vi "EasyFlux.vi"() -> ()   [LabVIEW 2017]
uses:
  Types/EF_GUIThread_SMCmds.ctl
  Types/EF_GUIThread_QData.ctl
  Types/EF_GUIThread_QCmds.ctl
  Types/EF_DAQThread_QData.ctl
  Types/EF_DAQThread_QCmds.ctl
  Types/EF_DataProcThread_QData.ctl
  Types/EF_DataProcThread_QCmds.ctl
  Types/EF_AnalysisThread_QData.ctl
  Types/EF_AnalysisThread_QCmds.ctl
panel:
  out "DeltaT":dbl caption="Resol.     ms" format="%.2f"
  in  "BitShift":i32 min=0 max=32 step=1
  in  "Threshold":i32 caption="Thresh. cnts" min=0 max=100000 step=1
  out "TimeChart":cluster{dbl, "DeltaT":dbl, u32[]}(graph)={0.0, "DeltaT"=0.0016383737860194236, []}
  in  "MinIntCounts":u32=1 caption="Min. Counts" min=1 step=1
  in  "DecayT0":dbl caption="DecayT0  ns" min=0.0 step=0.001
  in  "Offset":i32 caption="Offset      ps" min=0 max=100000 step=1
  in  "Binning":i32(ring) caption="Resol.      ps" items=["4", "8", "16", "32", "64", "128", "256", "512"]
  in  "CFD1 ZeroX":i32=10 caption="ZeroCr.  mV" min=0 max=20 step=1
  in  "CFD1 Level":i32=50 caption="Discr.     mV" min=0 max=800 step=1
  in  "Ch0 Divider":i32(ring)=1 caption="Divider" items=["1"=1, "2"=2, "4"=4, "8"=8]
  in  "Ch0 Offset":i32 caption="Offset      ps" min=-99999 max=99999 step=1
  in  "CFD0 ZeroX":i32=10 caption="ZeroCr.  mV" min=0 max=20 step=1
  in  "CFD0 Level":i32=50 caption="Discr.     mV" min=0 max=800 step=1
  out "HistoGraph":cluster{dbl, "Res":dbl, "Histo":u32[]}(graph)
  out "Pending":i32
  out "ShortDelay":bool caption="Short Delay"
  out "MinDelay":dbl(slide) caption="Minimum Delay             ms" scale=200.0..300.0 scale format="%#.0f"
  in  "LTThreshold":dbl caption="Thresh.    ns" min=0.0 step=0.001
  in  "Activate":bool
  in  "TTLWidth":i32=1 caption="Width     ms" min=1 max=10000 step=1
  in  "TTLDelay":i32=50 caption="Delay      ms" min=10 max=10000 step=1
  in  "Start":bool
  out "LTGraph":cluster{dbl[], "AvgLTs":dbl[]}(graph)
  out "Ch1 Rate:":i32 caption="Input1 / cps" format="%.2e"
  out "Ch0 Rate:":i32 caption="Sync / cps" format="%.2e"
  out "Status":string
  # "Time Trace"
  # "Histogram"
  # "Inp.Chan 1"
  # "Inp.Chan 0 / Sync"
  # "TTL Pulse"
  # "Lifetimes"
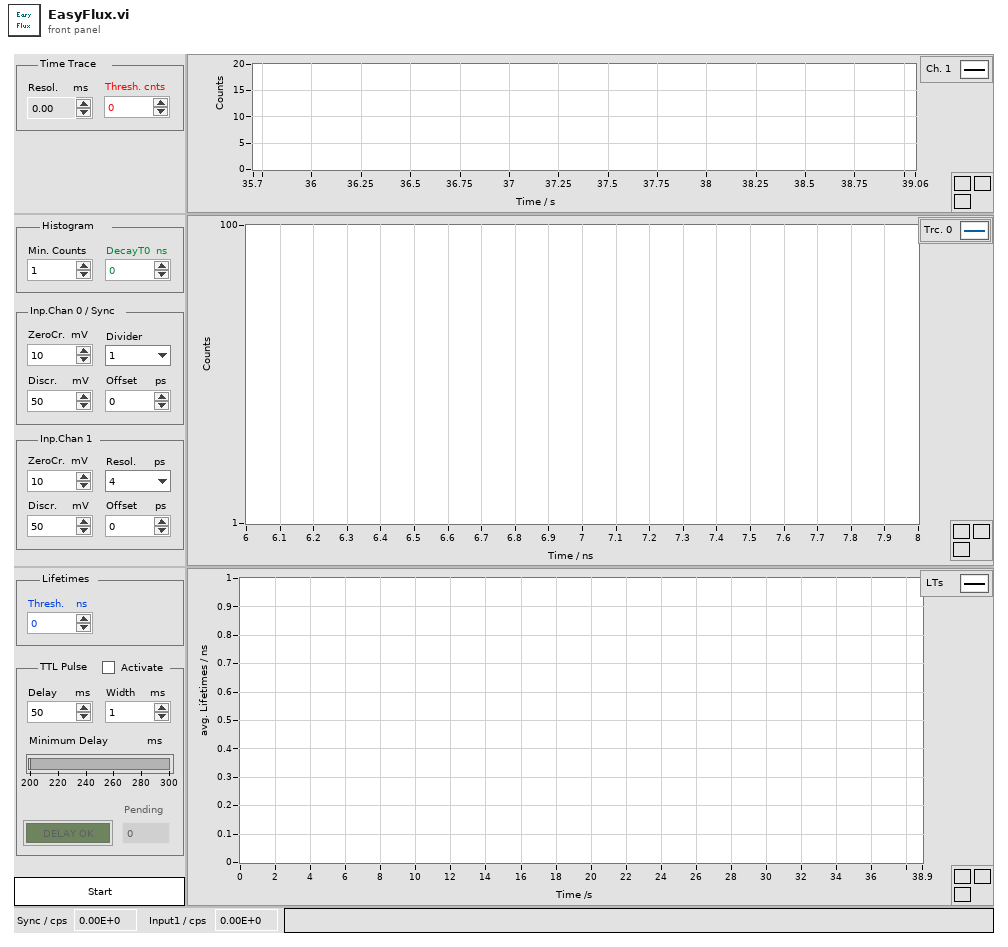
[diagram p1: front panel]
types:
  T1 = typedef "EF_GUIThread_QData.ctl" = cluster{"Histo":u32[], "Rates":i32[], "Cmd":T2, "Res":dbl, "TimeTrace":u32[], "Bin":i32, "Status":string, "Total bin":u64, "AvgLTs":dbl[], "TotalBinsHistStart":u64[], "HistStartTimes":dbl[], "MinDelays":dbl[], "ShortDelay":bool, "Pending TTLs":i32, "error in (no error)":errorcluster, "DeltaT":dbl, "NumLTs":i32}
  T2 = typedef "EF_GUIThread_QCmds.ctl" = enum16{"_none_", "Res", "Histo", "TTrace", "Lifetime", "Rates", "Status", "ShortDelay", "_Error_"}
  T3 = typedef "EF_GUIThread_SMCmds.ctl" = enum16{"Idle", "Enable Controls", "Init", "Timeout"}
  T4 = typedef "EF_GUIThread_IniData.ctl" = cluster{"Threshold":i32, "BitShift":i32, "DecayT0":dbl, "LTThreshold":dbl, "TTLDelay":i32, "TTLWidth":i32, "MinIntCounts":u32}
  T5 = typedef "EF_DAQThread_Data.ctl" = cluster{"LibraryVersion":string, "CFD0_Level":i32, "CFD0_ZeroX":i32, "CFD1_Level":i32, "CFD1_ZeroX":i32, "Ch0_Divider":i32, "Ch0_Offset":i32, "Init Info":T6, "DevIdx":i32, "Offset":i32, "Binning":i32, "Resolution":dbl, "DllPath":path, "Status":string}
  T6 = typedef "PH_InitInfo.ctl" = cluster{"Library Version":string, "Serial No.":string, "Model":string, "Partnum":string, "Version":string, "features":i32, "Base Resolution":dbl, "Bin Steps":i32, "DevIdx":i32}
  T7 = typedef "EF_AllQRefs.ctl" = cluster{"EF_GUIThread_QRef":T8, "EF_DAQThread_QRef":T9, "EF_DataProcThread_QRef":T10, "EF_AnalysisThread_QRef":T11}
  T8 = typedef "EF_GUIThread_QRef.ctl" = refnum<queue>
  T9 = typedef "EF_DAQThread_QRef.ctl" = refnum<queue>
  T10 = typedef "EF_DataProcThread_QRef.ctl" = refnum<queue>
  T11 = typedef "EF_AnalysisThread_QRef.ctl" = refnum<queue>
  T12 = typedef "EF_DAQThread_QData.ctl" = cluster{"EF_DAQThread_Cmds":T13, "Parameter":i32[], "error in (no error)":errorcluster}
  T13 = typedef "EF_DAQThread_QCmds.ctl" = enum16{"Idle", "Init", "InitHW", "SetCFD0", "SetCFD1", "SetCh0Divider", "SetCh0Offset", "SetOffset", "SetBinning", "GetResolution", "GetRates", "StartMeas", "ReadFiFo", "StopMeas", "WriteStatus", "_Error_", "Exit"}
  T14 = typedef "EF_DataProcThread_QCmds.ctl" = enum16{"Exit", "Proc", "Init", "SetShift", "SetThres"}
  T15 = typedef "EF_DataProcThread_QData.ctl" = cluster{"EF_DataProc_Cmds":T14, "nActual":i32, "Buffer":u32[], "TickCount":u32, "Param":i32}
  T16 = typedef "EF_AnalysisThread_QCmds.ctl" = enum16{"Exit", "CalcAvgLT", "CalcDelay", "SetDecayT0", "SetHistoRes", "SetTimeTraceRes", "SetLTThreshold", "SetTTLActiv", "SetTTLDelay", "SetTTLWidth", "SetMinIntCounts"}
  T17 = typedef "EF_AnalysisThread_QData.ctl" = cluster{"Cmd":T16, "Histo":u32[], "DecayT0":dbl, "HistoRes":dbl, "TotalBinHistStart":u64, "TimeTraceRes":dbl, "Total bin":u64, "TickCount":u32, "LTThreshold":dbl, "TTLActivate":bool, "TTLDelay":dbl, "TTLWidth":dbl, "MinIntCounts":u32}
  T18 = enum8{"Enabled", "Disabled", "Disabled and Grayed Out"}
  T19 = cluster{"T0":dbl, "dt":dbl, "TimeTrace_out":u32[]}
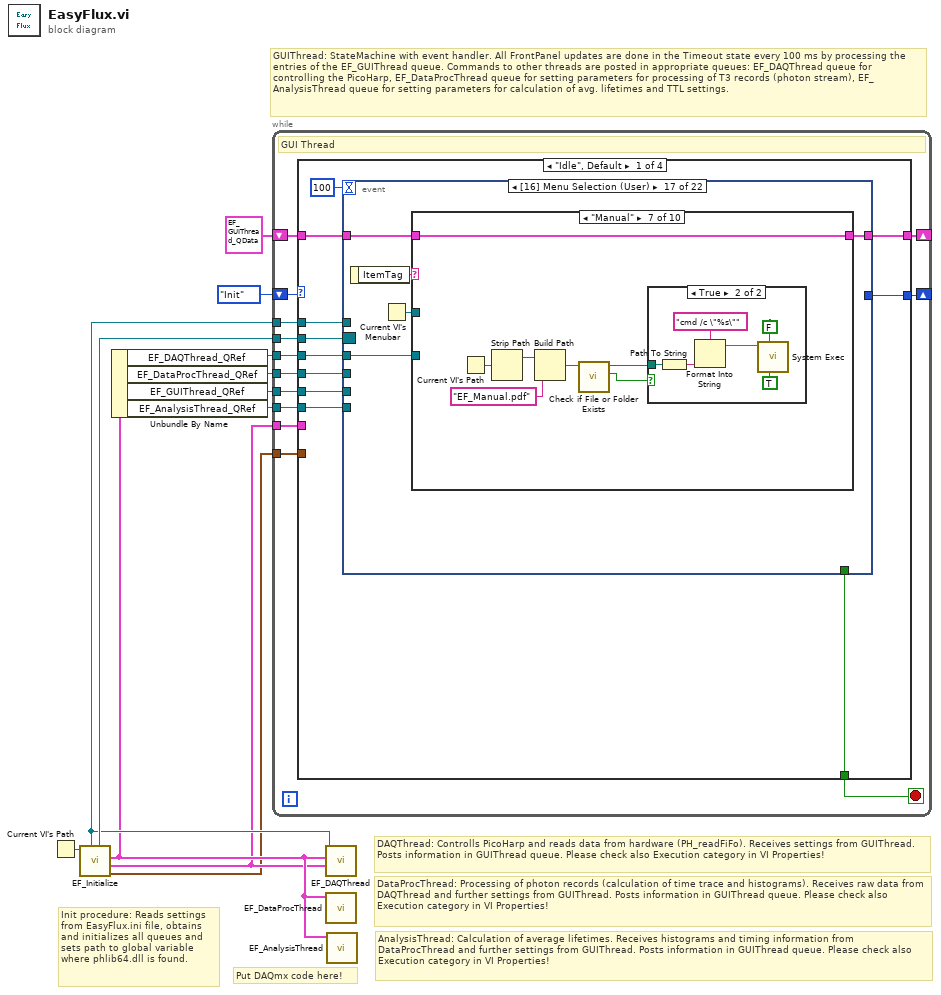
[diagram p0: block diagram]
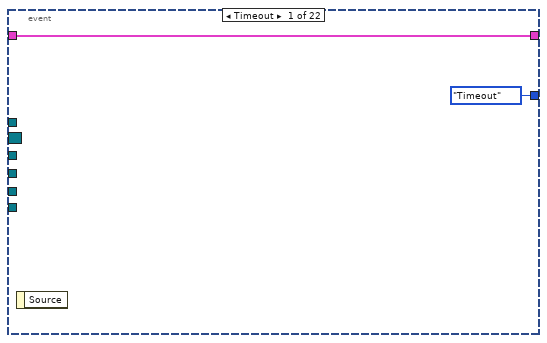
[diagram p2: hidden frame]
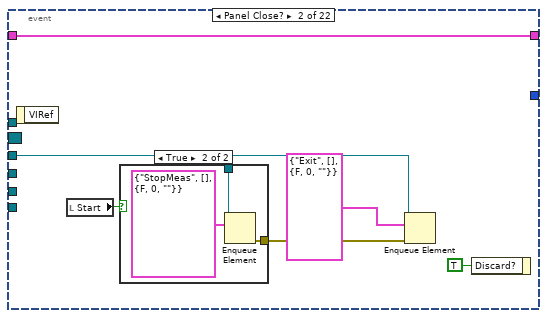
[diagram p3: hidden frame]
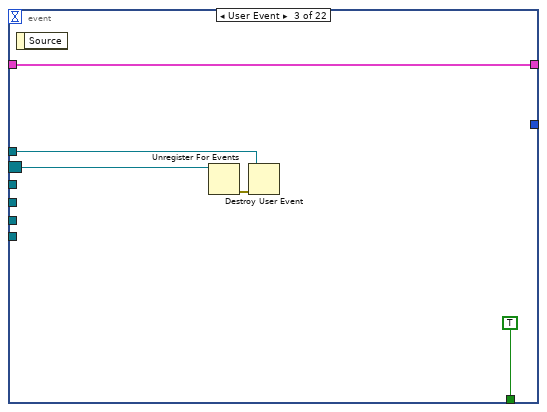
[diagram p5: hidden frame]
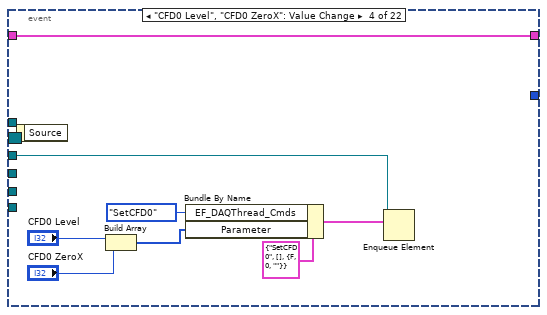
[diagram p6: hidden frame]
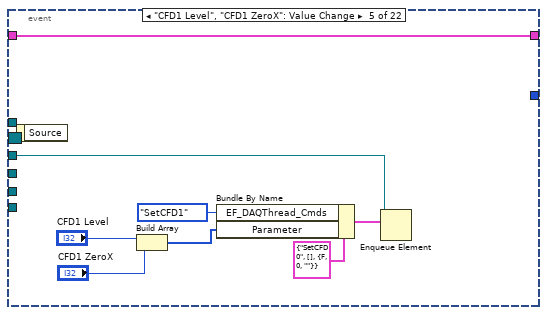
[diagram p7: hidden frame]
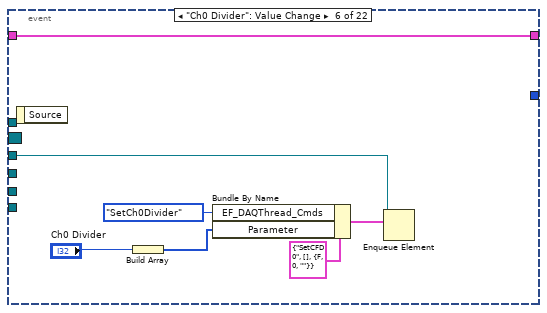
[diagram p8: hidden frame]
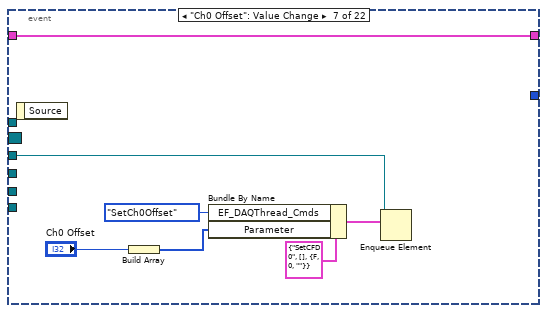
[diagram p9: hidden frame]
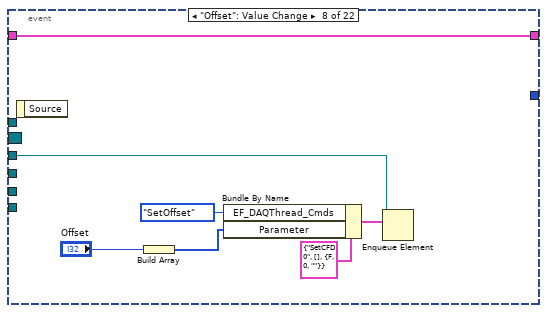
[diagram p10: hidden frame]
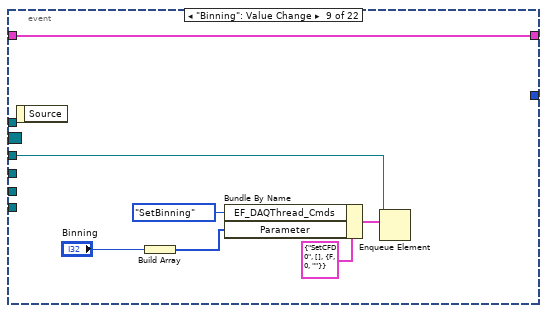
[diagram p11: hidden frame]
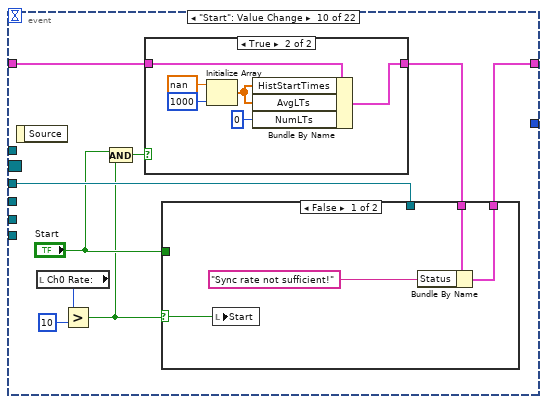
[diagram p12: hidden frame]
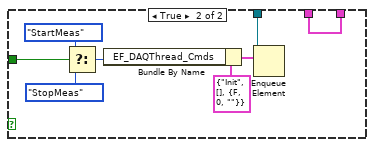
[diagram p13: hidden frame]
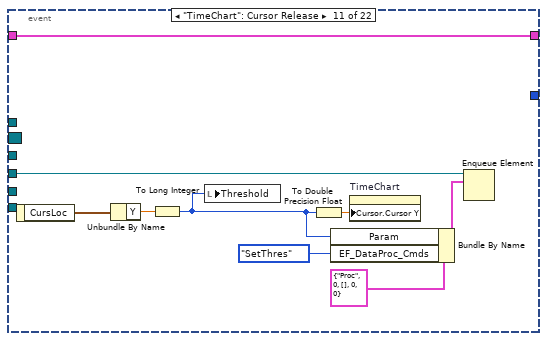
[diagram p15: hidden frame]
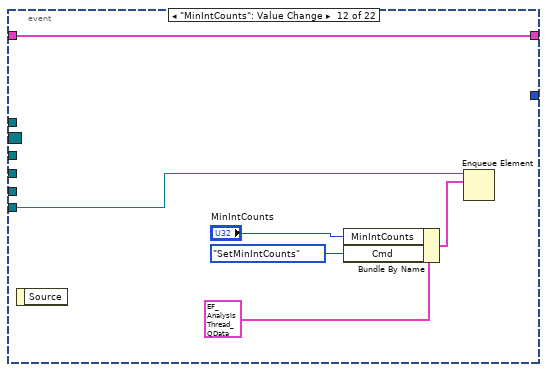
[diagram p16: hidden frame]
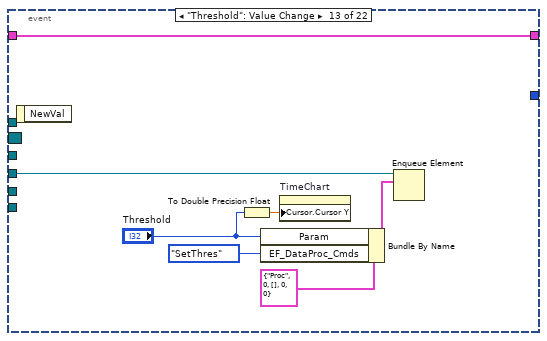
[diagram p17: hidden frame]
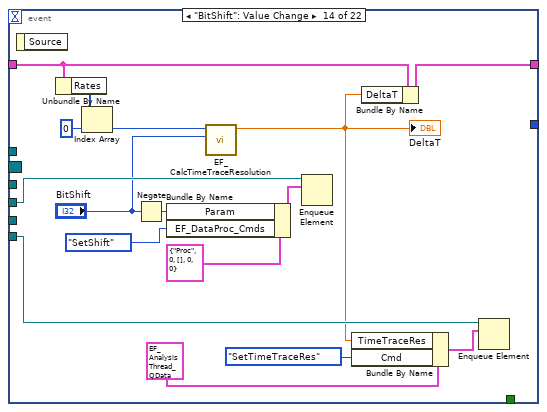
[diagram p18: hidden frame]
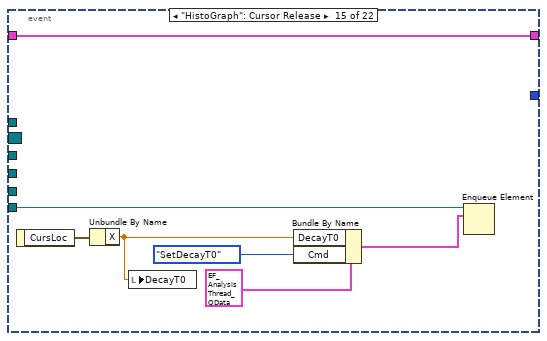
[diagram p19: hidden frame]
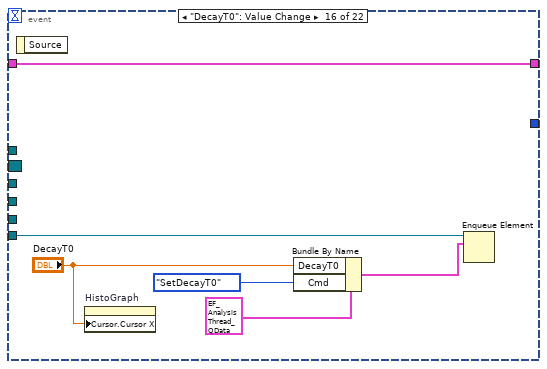
[diagram p20: hidden frame]
diagram:
  # "Init procedure: Reads settings from EasyFlux.ini file, obtains and initializes all queues and sets path to global variable where phlib64.dll is found."
  # "Put DAQmx code here!"
  # "DAQThread: Controlls PicoHarp and reads data from hardware (PH_readFiFo). Receives settings from GUIThread. Posts information in GUIThread queue. Please check also Execution category in VI Properties!"
  # "DataProcThread: Processing of photon records (calculation of time trace and histograms). Receives raw data from DAQThread and further settings from GUIThread. Posts information in GUIThread queue. Please check also Execution category in VI Properties!"
  # "GUIThread: StateMachine with event handler. All FrontPanel updates are done in the Timeout state every 100 ms by processing the entries of the EF_GUIThread queue. Commands to other threads are posted in appropriate queues: EF_DAQThread queue for controlling the PicoHarp, EF_DataProcThread queue for setting parameters for processing of T3 records (photon stream), EF_AnalysisThread queue for setting parameters for calculation of avg. lifetimes and TTL settings."
  # "AnalysisThread: Calculation of average lifetimes. Receives histograms and timing information from DataProcThread and further settings from GUIThread. Posts information in GUIThread queue. Please check also Execution category in VI Properties!"
  n1 = Current VI's Path() -> (path=w10:path)
  n2 = call "EF_Initialize.vi"("path"=w10) -> ("EF_DAQThread_IniData"=w1:T4, "EF_DAQThread_Data"=w2:T5, "EF_AllQRefs"=w3:T7, "ExitRef"=w9:refnum<event-registration>, "Exit"=w8:refnum<user-event>)  [unwired: 6 in]
  n3 = Unbundle By Name(w3) -> ("EF_DAQThread_QRef"=w7:T9, "EF_DataProcThread_QRef"=w6:T10, "EF_GUIThread_QRef"=w5:T8, "EF_AnalysisThread_QRef"=w4:T11)
  n4 = while {
    shift-right: [w17] -> _
    shift-left: EF_GUIThread_SMCmds."Init" -> [w25]
    tunnel: w7 -> [w24]
    tunnel: w9 -> [w23]
    tunnel: w5 -> [w21]
    tunnel: w6 -> [w20]
    shift-right: [w19] -> _
    shift-left: T1 {"Histo"=[], "Rates"=[], "Cmd"=enum."_none_", "Res"=0.0, "TimeTrace"=[], "Bin"=0, "Status"="", "Total bin"=0, "AvgLTs"=[], "TotalBinsHistStart"=[], "HistStartTimes"=[], "MinDelays"=[], "ShortDelay"=FALSE, "Pending TTLs"=0, "error in (no error)"={"status"=FALSE, "code"=0, "source"=""}, "DeltaT"=0.0, "NumLTs"=0} ("EF_VisualData") -> [w18]
    tunnel: w8 -> [w16]
    tunnel: w4 -> [w15]
    tunnel: w1 -> [w14]
    tunnel: w2 -> [w13]
    stop <- w22 stop-if-true
    # "GUI Thread"
    n5 = case shown="\"Idle\", Default" w25 {
      tunnel: w24 -> [w35 _ _ _]
      tunnel: [w28 w319 EF_GUIThread_SMCmds."Enable Controls" w390] -> w17
      tunnel: w23 -> [w34 _ _ _]
      tunnel: [w33 _ _ _] -> w22
      tunnel: w21 -> [w32 w320 _ _]
      tunnel: w20 -> [w31 _ _ _]
      tunnel: [w29 w296 w377 w394] -> w19
      tunnel: w18 -> [w30 w321 w375 w395]
      tunnel: w16 -> [w27 _ _ _]
      tunnel: w15 -> [w26 _ _ _]
      tunnel: w14 -> [_ _ w356 _]
      tunnel: w13 -> [_ _ w357 _]
      frame "Idle", Default {
        n6 = event shown="[16] Menu Selection (User)" {
          selector: w34 -> [_ _ w50 _ _ _ _ _ _ _ _ _ _ _ _ _ _ _ _ _ _ _]
          dyn-events: _ -> [_ _ _ _ _ _ _ _ _ _ _ _ _ _ _ _ _ _ _ _ _ _]
          timeout: 100 -> [_ _ _ _ _ _ _ _ _ _ _ _ _ _ _ _ _ _ _ _ _ _]
          tunnel: w35 -> [_ w41 _ w60 w68 w75 w82 w89 w96 w105 _ _ _ _ _ _ w177 _ _ _ _ _]
          tunnel: [_ _ TRUE _ _ _ _ _ _ _ _ _ _ _ _ _ _ _ _ _ _ _] -> w33
          tunnel: w32 -> [_ _ _ _ _ _ _ _ _ _ _ _ _ _ _ _ _ _ _ _ _ _]
          tunnel: w31 -> [_ _ _ _ _ _ _ _ _ _ w133 _ w142 w159 _ _ _ _ _ _ _ _]
          tunnel: w30 -> [w38 w39 w51 w53 w61 w69 w76 w83 w90 w104 w125 w139 w140 w148 w168 w175 w179 w259 w266 w275 w282 w289]
          tunnel: [w38 w39 w51 w53 w61 w69 w76 w83 w90 w97 w125 w139 w140 w149 w168 w175 w178 w259 w266 w275 w282 w289] -> w29
          tunnel: [EF_GUIThread_SMCmds."Timeout" _ _ _ _ _ _ _ _ _ _ _ _ _ _ _ _ _ _ _ _ _] -> w28
          tunnel: w27 -> [_ _ w48 _ _ _ _ _ _ _ _ _ _ _ _ _ _ _ _ _ _ _]
          tunnel: w26 -> [_ _ _ _ _ _ _ _ _ _ _ w137 _ w153 w167 w174 _ w258 w265 w274 w281 w288]
          event Timeout {
            n7 = event-data() -> ()  [unwired: 1 in, 1 out]
          }
          event Panel Close? {
            n8 = event-data() -> ()  [unwired: 1 in, 1 out]
            n9 = local read "Start"() -> (w42:bool)
            n10 = case shown="True" w42 {
              tunnel: w41 -> [_ w46]
              tunnel: [_ w45] -> w40
              frame False {
              }
              frame True {
                n11 = Enqueue Element(queue=w46, element=T12 {"EF_DAQThread_Cmds"=enum."StopMeas", "Parameter"=[], "error in (no error)"={"status"=FALSE, "code"=0, "source"=""}}) -> (error out=w45:errorcluster)  [unwired: 2 in, 2 out]
              }
            }
            n12 = Enqueue Element(queue=w41, element=T12 {"EF_DAQThread_Cmds"=enum."Exit", "Parameter"=[], "error in (no error)"={"status"=FALSE, "code"=0, "source"=""}}, error in (no error)=w40) -> ()  [unwired: 1 in, 3 out]
            n13 = event-data("Discard?"=TRUE) -> ()  [unwired: 1 in, 1 out]
          }
          event User Event {
            n14 = event-data() -> ()  [unwired: 1 in, 1 out]
            n15 = Unregister For Events(event registration refnum=w50) -> (error out=w49:errorcluster)  [unwired: 1 in]
            n16 = Destroy User Event(user event=w48, error in=w49) -> ()  [unwired: 1 out]
          }
          event "CFD0 Level", "CFD0 ZeroX": Value Change {
            n17 = event-data() -> ()  [unwired: 1 in, 1 out]
            n18 = Build Array("CFD0 Level", "CFD0 ZeroX") -> (w55:i32[])
            n19 = Bundle By Name(cluster=T12 {"EF_DAQThread_Cmds"=enum."SetCFD0", "Parameter"=[], "error in (no error)"={"status"=FALSE, "code"=0, "source"=""}} ("element"), "EF_DAQThread_Cmds"=EF_DAQThread_QCmds."SetCFD0", "Parameter"=w55) -> (w54:T12)
            n20 = Enqueue Element(queue=w60, element=w54) -> ()  [unwired: 2 in, 3 out]
          }
          event "CFD1 Level", "CFD1 ZeroX": Value Change {
            n21 = event-data() -> ()  [unwired: 1 in, 1 out]
            n22 = Build Array("CFD1 Level", "CFD1 ZeroX") -> (w65:i32[])
            n23 = Bundle By Name(cluster=T12 {"EF_DAQThread_Cmds"=enum."SetCFD0", "Parameter"=[], "error in (no error)"={"status"=FALSE, "code"=0, "source"=""}} ("element"), "EF_DAQThread_Cmds"=EF_DAQThread_QCmds."SetCFD1", "Parameter"=w65) -> (w64:T12)
            n24 = Enqueue Element(queue=w68, element=w64) -> ()  [unwired: 2 in, 3 out]
          }
          event "Ch0 Divider": Value Change {
            n25 = event-data() -> ()  [unwired: 1 in, 1 out]
            n26 = Build Array("Ch0 Divider") -> (w72:i32[])
            n27 = Bundle By Name(cluster=T12 {"EF_DAQThread_Cmds"=enum."SetCFD0", "Parameter"=[], "error in (no error)"={"status"=FALSE, "code"=0, "source"=""}} ("element"), "EF_DAQThread_Cmds"=EF_DAQThread_QCmds."SetCh0Divider", "Parameter"=w72) -> (w71:T12)
            n28 = Enqueue Element(queue=w75, element=w71) -> ()  [unwired: 2 in, 3 out]
          }
          event "Ch0 Offset": Value Change {
            n29 = event-data() -> ()  [unwired: 1 in, 1 out]
            n30 = Build Array("Ch0 Offset") -> (w79:i32[])
            n31 = Bundle By Name(cluster=T12 {"EF_DAQThread_Cmds"=enum."SetCFD0", "Parameter"=[], "error in (no error)"={"status"=FALSE, "code"=0, "source"=""}} ("element"), "EF_DAQThread_Cmds"=EF_DAQThread_QCmds."SetCh0Offset", "Parameter"=w79) -> (w78:T12)
            n32 = Enqueue Element(queue=w82, element=w78) -> ()  [unwired: 2 in, 3 out]
          }
          event "Offset": Value Change {
            n33 = event-data() -> ()  [unwired: 1 in, 1 out]
            n34 = Build Array("Offset") -> (w86:i32[])
            n35 = Bundle By Name(cluster=T12 {"EF_DAQThread_Cmds"=enum."SetCFD0", "Parameter"=[], "error in (no error)"={"status"=FALSE, "code"=0, "source"=""}} ("element"), "EF_DAQThread_Cmds"=EF_DAQThread_QCmds."SetOffset", "Parameter"=w86) -> (w85:T12)
            n36 = Enqueue Element(queue=w89, element=w85) -> ()  [unwired: 2 in, 3 out]
          }
          event "Binning": Value Change {
            n37 = event-data() -> ()  [unwired: 1 in, 1 out]
            n38 = Build Array("Binning") -> (w93:i32[])
            n39 = Bundle By Name(cluster=T12 {"EF_DAQThread_Cmds"=enum."SetCFD0", "Parameter"=[], "error in (no error)"={"status"=FALSE, "code"=0, "source"=""}} ("element"), "EF_DAQThread_Cmds"=EF_DAQThread_QCmds."SetBinning", "Parameter"=w93) -> (w92:T12)
            n40 = Enqueue Element(queue=w96, element=w92) -> ()  [unwired: 2 in, 3 out]
          }
          event "Start": Value Change {
            n41 = event-data() -> ()  [unwired: 1 in, 1 out]
            n42 = local read "Ch0 Rate:"() -> (w103:i32)
            n43 = Greater?(x=w103, y=10) -> (0:w99:bool)
            n44 = And(x="Start", y=w99) -> (x .and. y?=w100:bool)
            n45 = case shown="True" w100 {
              tunnel: w104 -> [w118 w124]
              tunnel: [w118 w123] -> w98
              frame False {
              }
              frame True {
                n46 = Initialize Array(nan ("element"), 1000 ("dimension size")) -> (w119:dbl[])
                n47 = Bundle By Name(cluster=w124, "HistStartTimes"=w119, "AvgLTs"=w119, "NumLTs"=0) -> (w123:T1)
              }
            }
            n48 = case shown="False" w99 {
              selector: w99 -> [w106 _]
              tunnel: w105 -> [_ w117]
              tunnel: "Start" -> [_ w111]
              tunnel: w98 -> [w109 w110]
              tunnel: [w108 w110] -> w97
              frame False {
                n49 = local write "Start"(w106) -> ()
                n50 = Bundle By Name(cluster=w109, "Status"="Sync rate not sufficient!") -> (w108:T1)
              }
              frame True {
                n51 = Select(t=EF_DAQThread_QCmds."StartMeas" ("EF_DAQThread_Cmds"), s=w111, f=EF_DAQThread_QCmds."StopMeas" ("EF_DAQThread_Cmds")) -> (s? t:f=w112:T13)
                n52 = Bundle By Name(cluster=T12 {"EF_DAQThread_Cmds"=enum."Init", "Parameter"=[], "error in (no error)"={"status"=FALSE, "code"=0, "source"=""}} ("element"), "EF_DAQThread_Cmds"=w112) -> (w115:T12)
                n53 = Enqueue Element(queue=w117, element=w115) -> ()  [unwired: 2 in, 3 out]
              }
            }
          }
          event "TimeChart": Cursor Release {
            n54 = event-data() -> ("CursLoc"=w130:cluster{"X":dbl, "Y":dbl})  [unwired: 1 in]
            n55 = Unbundle By Name(w130) -> ("Y"=w129:dbl)
            n56 = To Long Integer(number=w129) -> (32bit integer=w126:i32)
            n57 = local write "Threshold"(w126) -> ()
            n58 = To Double Precision Float(number=w126) -> (double precision float=w127:dbl)
            n59 = Bundle By Name(cluster=T15 {"EF_DataProc_Cmds"=enum."Proc", "nActual"=0, "Buffer"=[], "TickCount"=0, "Param"=0} ("element"), "Param"=w126, "EF_DataProc_Cmds"=EF_DataProcThread_QCmds."SetThres") -> (w128:T15)
            n60 = property on="TimeChart" class="WFGraph (strict)"("Cursor.Cursor Y"=w127) -> ()  [unwired: 2 in, 2 out]
            n61 = Enqueue Element(queue=w133, element=w128) -> ()  [unwired: 2 in, 3 out]
          }
          event "MinIntCounts": Value Change {
            n62 = event-data() -> ()  [unwired: 1 in, 1 out]
            n63 = Bundle By Name(cluster=T17 {"Cmd"=enum."Exit", "Histo"=[], "DecayT0"=0.0, "HistoRes"=0.0, "TotalBinHistStart"=0, "TimeTraceRes"=0.0, "Total bin"=0, "TickCount"=0, "LTThreshold"=0.0, "TTLActivate"=FALSE, "TTLDelay"=0.0, "TTLWidth"=0.0, "MinIntCounts"=0} ("element"), "MinIntCounts"="MinIntCounts", "Cmd"=EF_AnalysisThread_QCmds."SetMinIntCounts") -> (w134:T17)
            n64 = Enqueue Element(queue=w137, element=w134) -> ()  [unwired: 2 in, 3 out]
          }
          event "Threshold": Value Change {
            n65 = event-data() -> ()  [unwired: 1 in, 1 out]
            n66 = To Double Precision Float(number="Threshold") -> (double precision float=w145:dbl)
            n67 = Bundle By Name(cluster=T15 {"EF_DataProc_Cmds"=enum."Proc", "nActual"=0, "Buffer"=[], "TickCount"=0, "Param"=0} ("element"), "Param"="Threshold", "EF_DataProc_Cmds"=EF_DataProcThread_QCmds."SetThres") -> (w146:T15)
            n68 = property on="TimeChart" class="WFGraph (strict)"("Cursor.Cursor Y"=w145) -> ()  [unwired: 2 in, 2 out]
            n69 = Enqueue Element(queue=w142, element=w146) -> ()  [unwired: 2 in, 3 out]
          }
          event "BitShift": Value Change {
            n70 = event-data() -> ()  [unwired: 1 in, 1 out]
            n71 = Unbundle By Name(w148) -> ("Rates"=w158:i32[])
            n72 = Index Array(array=w158, index=0) -> (element=w154:i32)
            n73 = Negate(x="BitShift") -> (-x=w156:i32)
            n74 = Bundle By Name(cluster=T15 {"EF_DataProc_Cmds"=enum."Proc", "nActual"=0, "Buffer"=[], "TickCount"=0, "Param"=0} ("element"), "Param"=w156, "EF_DataProc_Cmds"=EF_DataProcThread_QCmds."SetShift") -> (w162:T15)
            n75 = call "EF_CalcTimeTraceResolution.vi"("BitShift"="BitShift", "Rate [Hz]"=w154) -> ("DeltaT [ms]"=w147:dbl)  [unwired: 9 in]
            "DeltaT" <- w147
            n76 = Enqueue Element(queue=w159, element=w162) -> ()  [unwired: 2 in, 3 out]
            n77 = Bundle By Name(cluster=T17 {"Cmd"=enum."Exit", "Histo"=[], "DecayT0"=0.0, "HistoRes"=0.0, "TotalBinHistStart"=0, "TimeTraceRes"=0.0, "Total bin"=0, "TickCount"=0, "LTThreshold"=0.0, "TTLActivate"=FALSE, "TTLDelay"=0.0, "TTLWidth"=0.0, "MinIntCounts"=0} ("element"), "TimeTraceRes"=w147, "Cmd"=EF_AnalysisThread_QCmds."SetTimeTraceRes") -> (w150:T17)
            n78 = Bundle By Name(cluster=w148, "DeltaT"=w147) -> (w149:T1)
            n79 = Enqueue Element(queue=w153, element=w150) -> ()  [unwired: 2 in, 3 out]
          }
          event "HistoGraph": Cursor Release {
            n80 = event-data() -> ("CursLoc"=w169:cluster{"X":dbl, "Y":dbl})  [unwired: 1 in]
            n81 = Unbundle By Name(w169) -> ("X"=w164:dbl)
            n82 = local write "DecayT0"(w164) -> ()
            n83 = Bundle By Name(cluster=T17 {"Cmd"=enum."Exit", "Histo"=[], "DecayT0"=0.0, "HistoRes"=0.0, "TotalBinHistStart"=0, "TimeTraceRes"=0.0, "Total bin"=0, "TickCount"=0, "LTThreshold"=0.0, "TTLActivate"=FALSE, "TTLDelay"=0.0, "TTLWidth"=0.0, "MinIntCounts"=0} ("element"), "DecayT0"=w164, "Cmd"=EF_AnalysisThread_QCmds."SetDecayT0" ("EF_AnalysisThread_Cmds")) -> (w163:T17)
            n84 = Enqueue Element(queue=w167, element=w163) -> ()  [unwired: 2 in, 3 out]
          }
          event "DecayT0": Value Change {
            n85 = event-data() -> ()  [unwired: 1 in, 1 out]
            n86 = property on="HistoGraph" class="WFGraph (strict)"("Cursor.Cursor X"="DecayT0") -> ()  [unwired: 2 in, 2 out]
            n87 = Bundle By Name(cluster=T17 {"Cmd"=enum."Exit", "Histo"=[], "DecayT0"=0.0, "HistoRes"=0.0, "TotalBinHistStart"=0, "TimeTraceRes"=0.0, "Total bin"=0, "TickCount"=0, "LTThreshold"=0.0, "TTLActivate"=FALSE, "TTLDelay"=0.0, "TTLWidth"=0.0, "MinIntCounts"=0} ("element"), "DecayT0"="DecayT0", "Cmd"=EF_AnalysisThread_QCmds."SetDecayT0" ("EF_AnalysisThread_Cmds")) -> (w171:T17)
            n88 = Enqueue Element(queue=w174, element=w171) -> ()  [unwired: 2 in, 3 out]
          }
          event Menu Selection (User) {
            n89 = event-data() -> ("ItemTag"=w180:string)  [unwired: 1 in]
            n90 = Current VI's Menubar() -> (w176:refnum<k9>)
            n91 = case shown="\"Manual\"" w180 {
              tunnel: w179 -> [w181 w183 w186 w189 w194 w208 w221 w236 w245 w254]
              tunnel: [w181 w182 w185 w188 w194 w208 w221 w236 w245 w254] -> w178
              tunnel: w177 -> [_ _ _ _ w195 _ _ _ _ _]
              tunnel: w176 -> [_ _ _ _ _ _ _ w235 w244 w253]
              frame Default {
              }
              frame "ClearTimeTrace" {
                n92 = in-place {
                  n93 = in-place-cluster #1(w183) -> ()  [unwired: 1 out]
                  n94 = in-place-cluster #1("TimeTrace"=u32[] []) -> (w182:T1)
                }
              }
              frame "ClearHisto" {
                n95 = in-place {
                  n96 = in-place-cluster #2(w186) -> ()  [unwired: 1 out]
                  n97 = in-place-cluster #2("Histo"=u32[] [] ("TimeTrace")) -> (w185:T1)
                }
              }
              frame "ClearLTGraph" {
                n98 = in-place {
                  n99 = in-place-cluster #3(w189) -> ()  [unwired: 3 out]
                  n100 = Initialize Array(nan ("element"), 1000 ("dimension size")) -> (w190:dbl[])
                  n101 = in-place-cluster #3("AvgLTs"=w190, "HistStartTimes"=w190, "NumLTs"=0) -> (w188:T1)
                }
              }
              frame "Exit" {
                n102 = local read "Start"() -> (w198:bool)
                n103 = case shown="True" w198 {
                  tunnel: w195 -> [_ w200]
                  tunnel: [_ w199] -> w197
                  frame False {
                  }
                  frame True {
                    n104 = Enqueue Element(queue=w200, element=T12 {"EF_DAQThread_Cmds"=enum."StopMeas", "Parameter"=[], "error in (no error)"={"status"=FALSE, "code"=0, "source"=""}}) -> (error out=w199:errorcluster)  [unwired: 2 in, 2 out]
                  }
                }
                n105 = Enqueue Element(queue=w195, element=T12 {"EF_DAQThread_Cmds"=enum."Exit", "Parameter"=[], "error in (no error)"={"status"=FALSE, "code"=0, "source"=""}}, error in (no error)=w197) -> ()  [unwired: 1 in, 3 out]
              }
              frame "OpenConfigFile" {
                n106 = Current VI's Path() -> (path=w206:path)
                n107 = Strip Path(path=w206) -> (stripped path=w205:path)  [unwired: 1 out]
                n108 = Build Path(base path=w205, name or relative path="EasyFlux.ini") -> (appended path=w207:path)
                n109 = call <vilib>:"Check if File or Folder Exists.vi"("path"=w207) -> ("file or folder exists?"=w203:bool, "dup path"=w204:path)  [unwired: 8 in, 1 out]
                n110 = case shown="True" w203 {
                  tunnel: w204 -> [_ w209]
                  frame False {
                  }
                  frame True {
                    n111 = Path To String(path=w209) -> (string=w213:string)
                    n112 = Format Into String(format string="cmd /c \"%s\"", w213) -> (resulting string=w214:string)  [unwired: 2 in, 1 out]
                    n113 = call <vilib>:"System Exec.vi"("run minimized? (F)"=TRUE, "wait until completion? (T)"=FALSE, "command line"=w214) -> ()  [unwired: 5 in, 4 out]
                  }
                }
              }
              frame "Manual" {
                n114 = Current VI's Path() -> (path=w219:path)
                n115 = Strip Path(path=w219) -> (stripped path=w218:path)  [unwired: 1 out]
                n116 = Build Path(base path=w218, name or relative path="EF_Manual.pdf") -> (appended path=w220:path)
                n117 = call <vilib>:"Check if File or Folder Exists.vi"("path"=w220) -> ("file or folder exists?"=w216:bool, "dup path"=w217:path)  [unwired: 8 in, 1 out]
                n118 = case shown="True" w216 {
                  tunnel: w217 -> [_ w222]
                  frame False {
                  }
                  frame True {
                    n119 = Path To String(path=w222) -> (string=w226:string)
                    n120 = Format Into String(format string="cmd /c \"%s\"", w226) -> (resulting string=w227:string)  [unwired: 2 in, 1 out]
                    n121 = call <vilib>:"System Exec.vi"("run minimized? (F)"=TRUE, "wait until completion? (T)"=FALSE, "command line"=w227) -> ()  [unwired: 5 in, 4 out]
                  }
                }
              }
              frame "LogTimeTrace" {
                w232 = "LogTimeTrace" ("item tag")
                n122 = Get Menu Item Info(7:w232, 11:w235) -> (3:w233:refnum<k9>, 4:w234:bool)  [unwired: 1 in, 5 out]
                n123 = Not(x=w234) -> (.not. x?=w231:bool)
                n124 = Set Menu Item Info(6:w231, 7:w232, 11:w233) -> ()  [unwired: 4 in, 2 out]
                n125 = Select(t=u8 1 ("Y Scale.Mapping Mode"), s=w231, f=u8 0 ("Y Scale.Mapping Mode")) -> (s? t:f=w228:u8)
                n126 = property on="TimeChart" class="WFGraph (strict)"("YScale.Mapping Mode"=w228) -> ()  [unwired: 2 in, 2 out]
              }
              frame "LogLTGraph" {
                w241 = "LogLTGraph" ("item tag")
                n127 = Get Menu Item Info(7:w241, 11:w244) -> (3:w242:refnum<k9>, 4:w243:bool)  [unwired: 1 in, 5 out]
                n128 = Not(x=w243) -> (.not. x?=w240:bool)
                n129 = Set Menu Item Info(6:w240, 7:w241, 11:w242) -> ()  [unwired: 4 in, 2 out]
                n130 = Select(t=u8 1 ("Y Scale.Mapping Mode"), s=w240, f=u8 0 ("Y Scale.Mapping Mode")) -> (s? t:f=w237:u8)
                n131 = property on="LTGraph" class="XYGraph (strict)"("YScale.Mapping Mode"=w237) -> ()  [unwired: 2 in, 2 out]
              }
              frame "LogHisto" {
                w250 = "LogHisto" ("item tag")
                n132 = Get Menu Item Info(7:w250, 11:w253) -> (3:w251:refnum<k9>, 4:w252:bool)  [unwired: 1 in, 5 out]
                n133 = Not(x=w252) -> (.not. x?=w249:bool)
                n134 = Set Menu Item Info(6:w249, 7:w250, 11:w251) -> ()  [unwired: 4 in, 2 out]
                n135 = Select(t=u8 1 ("Y Scale.Mapping Mode"), s=w249, f=u8 0 ("Y Scale.Mapping Mode")) -> (s? t:f=w246:u8)
                n136 = property on="HistoGraph" class="WFGraph (strict)"("YScale.Mapping Mode"=w246) -> ()  [unwired: 2 in, 2 out]
              }
            }
          }
          event "LTGraph": Cursor Release {
            n137 = event-data() -> ("CursLoc"=w261:cluster{"X":dbl, "Y":dbl})  [unwired: 1 in]
            n138 = Unbundle By Name(w261) -> ("Y"=w255:dbl)
            n139 = local write "LTThreshold"(w255) -> ()
            n140 = Bundle By Name(cluster=T17 {"Cmd"=enum."Exit", "Histo"=[], "DecayT0"=0.0, "HistoRes"=0.0, "TotalBinHistStart"=0, "TimeTraceRes"=0.0, "Total bin"=0, "TickCount"=0, "LTThreshold"=0.0, "TTLActivate"=FALSE, "TTLDelay"=0.0, "TTLWidth"=0.0, "MinIntCounts"=0} ("element"), "LTThreshold"=w255, "Cmd"=EF_AnalysisThread_QCmds."SetLTThreshold") -> (w260:T17)
            n141 = Enqueue Element(queue=w258, element=w260) -> ()  [unwired: 2 in, 3 out]
          }
          event "LTThreshold": Value Change {
            n142 = event-data() -> ()  [unwired: 1 in, 1 out]
            n143 = property on="LTGraph" class="XYGraph (strict)"("Cursor.Cursor Y"="LTThreshold") -> ()  [unwired: 2 in, 2 out]
            n144 = Bundle By Name(cluster=T17 {"Cmd"=enum."Exit", "Histo"=[], "DecayT0"=0.0, "HistoRes"=0.0, "TotalBinHistStart"=0, "TimeTraceRes"=0.0, "Total bin"=0, "TickCount"=0, "LTThreshold"=0.0, "TTLActivate"=FALSE, "TTLDelay"=0.0, "TTLWidth"=0.0, "MinIntCounts"=0} ("element"), "LTThreshold"="LTThreshold", "Cmd"=EF_AnalysisThread_QCmds."SetLTThreshold") -> (w267:T17)
            n145 = Enqueue Element(queue=w265, element=w267) -> ()  [unwired: 2 in, 3 out]
          }
          event "Activate": Value Change {
            n146 = event-data() -> ()  [unwired: 1 in, 1 out]
            n147 = Select(t=T18."Enabled" ("Disabled"), s="Activate", f=T18."Disabled and Grayed Out" ("Disabled")) -> (s? t:f=w268:T18)
            n148 = property on="ShortDelay" class="Bool (strict)"("DisabledEnum"=w268) -> ()  [unwired: 2 in, 2 out]
            n149 = property on="Pending" class="DigNum (strict)"("DisabledEnum"=w268) -> ()  [unwired: 2 in, 2 out]
            n150 = Bundle By Name(cluster=T17 {"Cmd"=enum."Exit", "Histo"=[], "DecayT0"=0.0, "HistoRes"=0.0, "TotalBinHistStart"=0, "TimeTraceRes"=0.0, "Total bin"=0, "TickCount"=0, "LTThreshold"=0.0, "TTLActivate"=FALSE, "TTLDelay"=0.0, "TTLWidth"=0.0, "MinIntCounts"=0} ("element"), "TTLActivate"="Activate", "Cmd"=EF_AnalysisThread_QCmds."SetTTLActiv") -> (w276:T17)
            n151 = Enqueue Element(queue=w274, element=w276) -> ()  [unwired: 2 in, 3 out]
          }
          event "TTLDelay": Value Change {
            n152 = event-data() -> ()  [unwired: 1 in, 3 out]
            n153 = To Double Precision Float(number="TTLDelay") -> (double precision float=w278:dbl)
            n154 = Bundle By Name(cluster=T17 {"Cmd"=enum."Exit", "Histo"=[], "DecayT0"=0.0, "HistoRes"=0.0, "TotalBinHistStart"=0, "TimeTraceRes"=0.0, "Total bin"=0, "TickCount"=0, "LTThreshold"=0.0, "TTLActivate"=FALSE, "TTLDelay"=0.0, "TTLWidth"=0.0, "MinIntCounts"=0} ("element"), "TTLDelay"=w278, "Cmd"=EF_AnalysisThread_QCmds."SetTTLDelay") -> (w283:T17)
            n155 = Enqueue Element(queue=w281, element=w283) -> ()  [unwired: 2 in, 3 out]
          }
          event "TTLWidth": Value Change {
            n156 = event-data() -> ()  [unwired: 1 in, 3 out]
            n157 = To Double Precision Float(number="TTLWidth") -> (double precision float=w285:dbl)
            n158 = Bundle By Name(cluster=T17 {"Cmd"=enum."Exit", "Histo"=[], "DecayT0"=0.0, "HistoRes"=0.0, "TotalBinHistStart"=0, "TimeTraceRes"=0.0, "Total bin"=0, "TickCount"=0, "LTThreshold"=0.0, "TTLActivate"=FALSE, "TTLDelay"=0.0, "TTLWidth"=0.0, "MinIntCounts"=0} ("element"), "TTLWidth"=w285, "Cmd"=EF_AnalysisThread_QCmds."SetTTLWidth") -> (w290:T17)
            n159 = Enqueue Element(queue=w288, element=w290) -> ()  [unwired: 2 in, 3 out]
          }
        }
      }
      frame "Timeout" {
        n160 = Flush Queue(queue=w320) -> (remaining elements=w338:T1[])  [unwired: 1 in, 2 out]
        n161 = Array Size(array=w338) -> (size(s)=w337:i32)
        n162 = Not Equal To 0?(x=w337) -> (x != 0?=w336:bool)
        n163 = case shown="True" w336 {
          tunnel: w338 -> [_ w348]
          tunnel: w321 -> [w343 w347]
          tunnel: [w343 w346] -> w296
          tunnel: [_ w345] -> w293
          tunnel: [_ w344] -> w292
          frame False {
          }
          frame True {
            n164 = call "EF_ReadVisualDataQ.vi"("EF_GUIThread_QDataList"=w348, "EF_GUIThread_QData"=w347) -> ("Error"=w344:errorcluster, "EF_GUIThread_QData_out"=w346:T1, "isError"=w345:bool)  [unwired: 7 in]
          }
        }
        n165 = Unbundle By Name(w296) -> ("Status"=w295:string, "Rates"=w335:i32[], "Res"=w330:dbl, "Histo"=w333:u32[], "DeltaT"=w291:dbl, "Total bin"=w317:u64, "Bin"=w316:i32, "TimeTrace"=w315:u32[], "HistStartTimes"=w307:dbl[], "AvgLTs"=w309:dbl[], "MinDelays"=w302:dbl[], "ShortDelay"=→"ShortDelay":bool, "Pending TTLs"=→"Pending":i32)
        "Status" <- w295
        n166 = case shown="True" w293 {
          tunnel: w292 -> [_ w339]
          frame False {
          }
          frame True {
            n167 = call <vilib>:"Simple Error Handler.vi"("error in (no error)"=w339) -> ()  [unwired: 4 in, 5 out]
            n168 = local write "Start"(FALSE ("Start")) -> ()
          }
        }
        n169 = property on="MinDelay" class="Slide (strict)"() -> ("Scale.Maximum"=w301:dbl, "Scale.Minimum"=w300:dbl)  [unwired: 2 in, 2 out]
        n170 = call "EF_CalcMinDelay.vi"("MinDelays"=w302, "Scale.Minimum in"=w300, "Scale.Maximum in"=w301) -> ("Scale.Minimum out"=w299:dbl, "rescale"=w298:bool, "Scale.Maximum out"=w303:dbl)  [unwired: 6 in]
        n171 = case shown="True" w298 {
          tunnel: w303 -> [_ w342]
          tunnel: w299 -> [_ w341]
          frame False {
          }
          frame True {
            n172 = property on="MinDelay" class="Slide (strict)"("Scale.Maximum"=w342, "Scale.Minimum"=w341) -> ()  [unwired: 2 in, 2 out]
          }
        }
        n173 = Divide(x=w330, y=1000.0) -> (x/y=w329:dbl)
        n174 = Index Array(array=w335, index #1=0 ("index"), index #2=1 ("index")) -> (element #1=w312:i32, element #2=→"Ch1 Rate:":i32)
        "Ch0 Rate:" <- w312
        n175 = local read "BitShift"() -> (w311:i32)
        n176 = call "EF_CalcTimeTrace.vi"("DeltaT"=w291, "TimeTrace"=w315, "Bin"=w316, "Total bin"=w317) -> ("TimeTrace_out"=w314:u32[], "dt"=w310:dbl, "T0"=w313:dbl)  [unwired: 5 in]
        n177 = Equal?(x="Init done.", y=w295) -> (x = y?=w331:bool)
        n178 = Bundle(0.0, w329, "Histo"=w333) -> (→"HistoGraph":cluster{dbl, dbl, "Histo":u32[]})  [unwired: 1 in]
        n179 = call "EF_CalcTimeTraceResolution.vi"("BitShift"=w311, "Rate [Hz]"=w312) -> ("DeltaT [ms]"=w306:dbl)  [unwired: 9 in]
        n180 = Bundle("HistStartTimes"=w307, "AvgLTs"=w309) -> (→"LTGraph":cluster{"HistStartTimes":dbl[], "AvgLTs":dbl[]})  [unwired: 1 in]
        n181 = Bundle("T0"=w313, "dt"=w310, "TimeTrace_out"=w314) -> (→"TimeChart":T19)  [unwired: 1 in]
        n182 = Select(t=EF_GUIThread_SMCmds."Enable Controls", s=w331, f=EF_GUIThread_SMCmds."Idle") -> (s? t:f=w319:T3)
        n183 = Index Array(array=w302, index=1) -> (element=→"MinDelay":dbl)
        n184 = local write "DeltaT"(w306) -> ()
      }
      frame "Init" {
        n185 = Initialize Array(250.0 ("element"), 10 ("dimension size")) -> (w363:dbl[])
        n186 = Bundle By Name(cluster=w375, "Status"="Initializing...", "MinDelays"=w363) -> (w377:T1)
        n187 = Unbundle By Name(w356) -> ("Threshold"=w355:i32, "BitShift"=w354:i32, "DecayT0"=w353:dbl, "LTThreshold"=w352:dbl, "TTLDelay"=w351:i32, "TTLWidth"=w350:i32, "MinIntCounts"=w349:u32)
        n188 = Unbundle By Name(w357) -> ("CFD0_Level"=w386:i32, "CFD0_ZeroX"=w385:i32, "CFD1_Level"=w384:i32, "CFD1_ZeroX"=w383:i32, "Ch0_Divider"=w382:i32, "Ch0_Offset"=w381:i32, "Offset"=w380:i32, "Binning"=w379:i32)
        n189 = property on="TimeChart" class="WFGraph (strict)"("YScale.Mapping Mode"=u8 0 ("Y Scale.Mapping Mode"), "XScale.ScaleFit"=u8 2 ("X Scale.Scale Fit")) -> ()  [unwired: 2 in, 2 out]
        n190 = local write "CFD0 Level"(w386) -> ()
        n191 = local write "CFD0 ZeroX"(w385) -> ()
        n192 = local write "CFD1 Level"(w384) -> ()
        n193 = local write "CFD1 ZeroX"(w383) -> ()
        n194 = local write "Ch0 Divider"(w382) -> ()
        n195 = local write "Ch0 Offset"(w381) -> ()
        n196 = local write "Offset"(w380) -> ()
        n197 = local write "Binning"(w379) -> ()
        n198 = local write "Threshold"(w355) -> ()
        n199 = local write "BitShift"(w354) -> ()
        n200 = local write "DecayT0"(w353) -> ()
        n201 = local write "LTThreshold"(w352) -> ()
        n202 = local write "TTLDelay"(w351) -> ()
        n203 = local write "TTLWidth"(w350) -> ()
        n204 = local write "MinIntCounts"(w349) -> ()
        n205 = property on="LTGraph" class="XYGraph (strict)"("YScale.Mapping Mode"=u8 0 ("Y Scale.Mapping Mode")) -> ()  [unwired: 2 in, 2 out]
        n206 = property on="MinDelay" class="Slide (strict)"("Scale.Maximum"=300.0 ("Scale.Range:Maximum"), "Scale.Minimum"=200.0 ("Scale.Range:Minimum")) -> ()  [unwired: 2 in, 2 out]
        n207 = Current VI's Menubar() -> (w374:refnum<k9>)
        n208 = Set Menu Item Info(6:FALSE ("checked"), 7:"LogTimeTrace" ("item tag"), 11:w374) -> ()  [unwired: 4 in, 2 out]
        n209 = Set Menu Item Info(6:FALSE ("checked"), 7:"LogLTGraph" ("item tag"), 11:w374) -> ()  [unwired: 4 in, 2 out]
        n210 = Set Menu Item Info(6:TRUE ("checked"), 7:"LogHisto" ("item tag"), 11:w374) -> ()  [unwired: 4 in, 2 out]
        n211 = property on="HistoGraph" class="WFGraph (strict)"("YScale.Mapping Mode"=u8 1 ("Y Scale.Mapping Mode")) -> ()  [unwired: 2 in, 2 out]
        n212 = local write "Start"(FALSE ("Start")) -> ()
        n213 = local write "Activate"(FALSE ("Activate")) -> ()
      }
      frame "Enable Controls" {
        w388 = T18."Disabled and Grayed Out" ("Disabled")
        n214 = Unbundle By Name(w395) -> ("Status"=w397:string)
        n215 = case shown="\"Init done.\"" w397 {
          tunnel: [T18."Enabled" ("Disabled") T18."Disabled and Grayed Out" ("Disabled")] -> w396
          tunnel: w395 -> [w412 w416]
          tunnel: [w411 w416] -> w394
          tunnel: [TRUE _] -> w391
          tunnel: [EF_GUIThread_SMCmds."Timeout" EF_GUIThread_SMCmds."Idle"] -> w390
          frame "Init done." {
            n216 = local read "Threshold"() -> (w408:i32)
            n217 = local read "BitShift"() -> (w407:i32)
            n218 = local read "DecayT0"() -> (w405:dbl)
            n219 = local read "LTThreshold"() -> (w404:dbl)
            n220 = local read "TTLDelay"() -> (w403:i32)
            n221 = local read "TTLWidth"() -> (w402:i32)
            n222 = local read "MinIntCounts"() -> (w401:u32)
            n223 = Bundle By Name(cluster=w412, "Status"="Initialized") -> (w411:T1)
            n224 = property on="Threshold" class="DigNum (strict)"("Val(Sgnl)"=w408) -> ()  [unwired: 2 in, 2 out]
            n225 = property on="BitShift" class="DigNum (strict)"("Val(Sgnl)"=w407) -> ()  [unwired: 2 in, 2 out]
            n226 = property on="DecayT0" class="DigNum (strict)"("Val(Sgnl)"=w405) -> ()  [unwired: 2 in, 2 out]
            n227 = property on="LTThreshold" class="DigNum (strict)"("Val(Sgnl)"=w404) -> ()  [unwired: 2 in, 2 out]
            n228 = property on="TTLDelay" class="DigNum (strict)"("Val(Sgnl)"=w403) -> ()  [unwired: 2 in, 2 out]
            n229 = property on="TTLWidth" class="DigNum (strict)"("Val(Sgnl)"=w402) -> ()  [unwired: 2 in, 2 out]
            n230 = property on="MinIntCounts" class="DigNum (strict)"("Val(Sgnl)"=w401) -> ()  [unwired: 2 in, 2 out]
          }
          frame "Initializing...", Default {
          }
        }
        n231 = property class="VI"() -> ("Panel"=w393:refnum<vi>)  [unwired: 2 in, 2 out]
        n232 = property class="Pnl"(reference=w393) -> ("Decos[]"=w392:refnum<vi>[])  [unwired: 1 in, 2 out]
        n233 = property class="Pnl"(reference=w393) -> ("Controls[]"=w398:refnum<vi>[])  [unwired: 1 in, 2 out]
        n234 = for {
          tunnel: w392 -> [w400] mode=indexing
          tunnel: w391 -> [w399]
          n235 = property class="Decor"(reference=w400, "Visible"=w399) -> ()  [unwired: 1 in, 2 out]
        }
        n236 = for {
          tunnel: w398 -> [w419] mode=indexing
          tunnel: w396 -> [w418]
          tunnel: [w417] -> w389
          n237 = property class="Ctl"(reference=w419, "DisabledEnum"=w418) -> (error out=w417:errorcluster)  [unwired: 1 in, 1 out]
        }
        n238 = property on="ShortDelay" class="Bool (strict)"(error in=w389, "DisabledEnum"=w388) -> ()  [unwired: 1 in, 2 out]
        n239 = property on="Pending" class="DigNum (strict)"(error in=w389, "DisabledEnum"=w388) -> ()  [unwired: 1 in, 2 out]
      }
    }
  }
  n240 = call "EF_DAQThread.vi"("EF_DAQThread_Data"=w2, "EF_AllQRefs"=w3, "Exit"=w8) -> ()  [unwired: 9 in]
  n241 = call "EF_DataProcThread.vi"("EF_AllQRefs"=w3) -> ()  [unwired: 11 in]
  n242 = call "EF_AnalysisThread.vi"("EF_AllQRefs"=w3) -> ()  [unwired: 11 in]
